vi "daqio_Create_Device_Type.vi"(6 "Device Type Label":string="Device Type Label", 7 "Device Type Key":string="LABVIEW_DEVICE_TYPE", 8 "error in (no error)":errorcluster, 11 "daq.io type in":T1={"daq.io ref"=refnum, "daq.io API Base"="http://dashboard.daq.io/api/v1", "Device Type Key"="", "Device Key"="", "Account ID"=""}) -> (0 "error out":errorcluster, 3 "daq.io type out":T1={"daq.io ref"=refnum, "daq.io API Base"="http://dashboard.daq.io/api/v1", "Device Type Key"="", "Device Key"="", "Account ID"=""})   [LabVIEW 2013, in "daqio minimal.lvlib"]
doc: "This VI creates a new device type that will act as a template for any number of new devices of the same type. The device type defines which events, tags and channels a device provides."
uses:
  daqio minimal.lvlib
  <vilib>/Easy HTTP Client/HTTP Header.ctl
  _typedefs/daqio-Type.ctl
  <vilib>/httpClient/ClientHandle.ctl
  <vilib>/Easy HTTP Client/Easy HTTP.lvlib
  <vilib>/httpClient/LabVIEWHTTPClient.lvlib
panel:
  out "JSON string":string
  out "headers":T3[](array[typedef])
  out "body":string
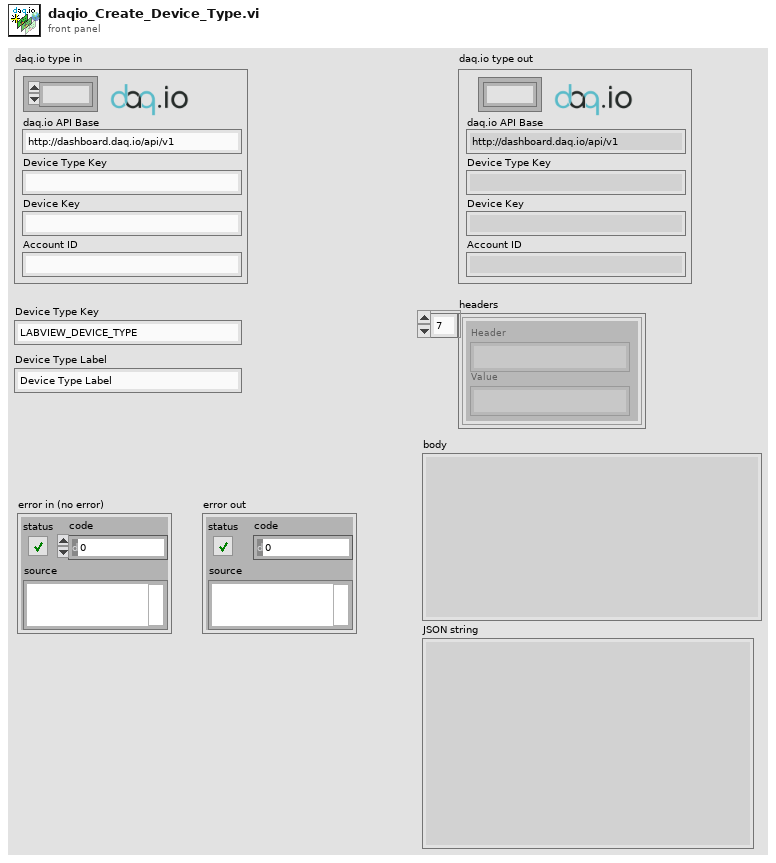
[diagram p1: front panel]
types:
  T1 = typedef "daqio minimal.lvlib/daqio-Type.ctl" = cluster{"daq.io ref":T2, "daq.io API Base":string, "Device Type Key":string, "Device Key":string, "Account ID":string}
  T2 = typedef "LabVIEWHTTPClient.lvlib/ClientHandle.ctl" = refnum<k1>
  T3 = typedef "Easy HTTP.lvlib/HTTP Header.ctl" = cluster{"Header":string, "Value":string}
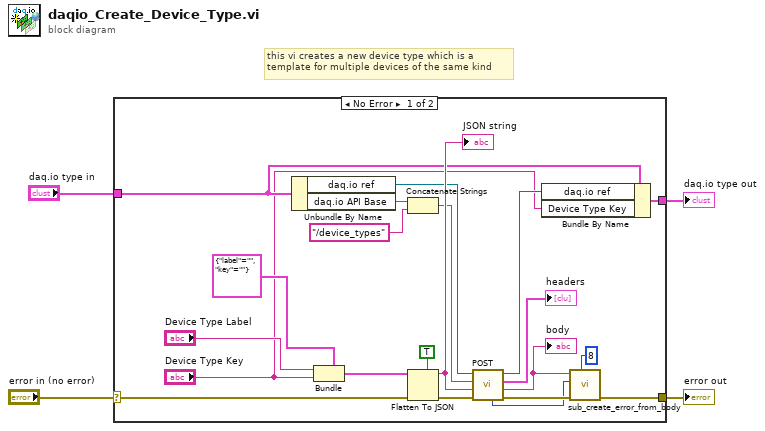
[diagram p0: block diagram]
diagram:
  # "this vi creates a new device type which is a \ntemplate for multiple devices of the same kind"
  n1 = case shown="No Error" "error in (no error)" {
    selector: "error in (no error)" -> [w9 w26]
    tunnel: "daq.io type in" -> [w17 w27]
    tunnel: [w15 w27] -> w3
    tunnel: [w11 w26] -> w2
    frame No Error {
      n2 = Unbundle By Name(w17) -> ("daq.io ref"=w18:T2, "daq.io API Base"=w14:string)
      n3 = Bundle(cluster=cluster{"label":string, "key":string} {"label"="", "key"=""}, "label"="Device Type Label", "key"="Device Type Key") -> (w24:cluster{"label":string, "key":string})
      n4 = Concatenate Strings(w14, "/device_types") -> (w21:string)
      n5 = Flatten To JSON(enable LabVIEW extensions? (T)=TRUE, anything=w24, error in (no error)=w9) -> (JSON string=w22:string, 11:w25:errorcluster)
      "JSON string" <- w22
      n6 = call <vilib>:"POST.vi"("error in (no error)"=w25, "data"=w22, "url"=w21, "client handle"=w18) -> ("error out"=w13:errorcluster, "body"=w12:string, "headers"=→"headers":T3[], "client handle out"=w16:T2, "HTTP Response Code"=w6:i32)  [unwired: 3 in]
      "body" <- w12
      n7 = Bundle By Name(cluster=w17, "daq.io ref"=w16, "Device Type Key"="Device Type Key") -> (w15:T1)
      n8 = call "sub_create_error_from_body.vi"("error code"=8, "error in (no error)"=w13, "http code"=w6, "body"=w12) -> ("error out"=w11:errorcluster)  [unwired: 7 in]
    }
    frame Error {
    }
  }
  "error out" <- w2
  "daq.io type out" <- w3
